vi "60MFile 읽기.vi"() -> ()   [LabVIEW 2014]
uses:
  <vilib>/Utility/file.llb/Read From Spreadsheet File (DBL).vi
panel:
  out "first row":dbl[](array[numeric]) caption="첫번째 행" format="%0.3f"
  in  "file path (dialog if empty)":path caption="파일 경로(비었을 경우 대화 상자)"
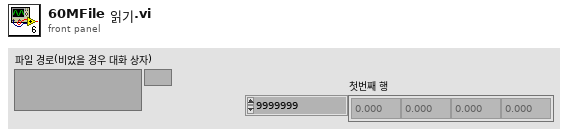
[diagram p1: front panel]
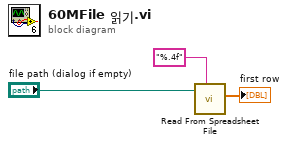
[diagram p0: block diagram]
diagram:
  n1 = call-poly <vilib>:"Read From Spreadsheet File.vi"("format (%.3f)"="%.4f", "file path (dialog if empty)"="file path (dialog if empty)") -> ("first row"=→"first row":dbl[])  [unwired: 5 in, 4 out]
